vi "Read Connection ID.vi"(11 "TCP Stream in":refnum<class "TCP Stream.lvclass">) -> (2 "connection ID":refnum<k5>)   [LabVIEW 2020, in "TCP Stream.lvclass"]
uses:
  TCP Stream.lvclass
  TCP Stream.lvclass/TCP Stream.ctl
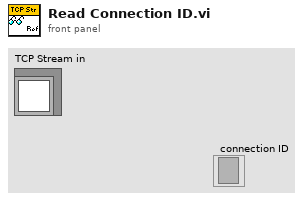
[diagram p1: front panel]
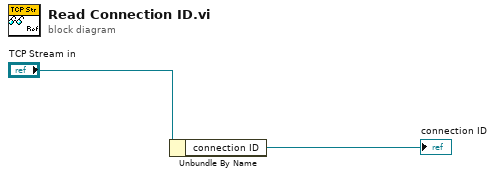
[diagram p0: block diagram]
diagram:
  n1 = Unbundle By Name("TCP Stream in") -> ("connection ID"=→"connection ID":refnum<k5>)
